vi "Add Data Type.vi"(7 "Control Info Cluster in":T1, 8 "error in (no error)":errorcluster, 10 "Data Type String":string, 11 "Control in":refnum<vi>) -> (0 "error out":errorcluster, 2 "TypeDef?":bool, 3 "Control out":refnum<vi>, 5 "Control Info Cluster out":T1)   [LabVIEW 2023, in "VIDoc Parsing.lvlib"]
doc: "Adds Data Type String to the Control Info Cluster, handing Typedefs specially."
uses:
  VIDoc Parsing.lvlib
  TypeDefs/Controls Info Cluster.ctl
  <vilib>/picture/picture.llb/imagedata.ctl
  <vilib>/Utility/miscctls.llb/LVKeyTypeDef.ctl
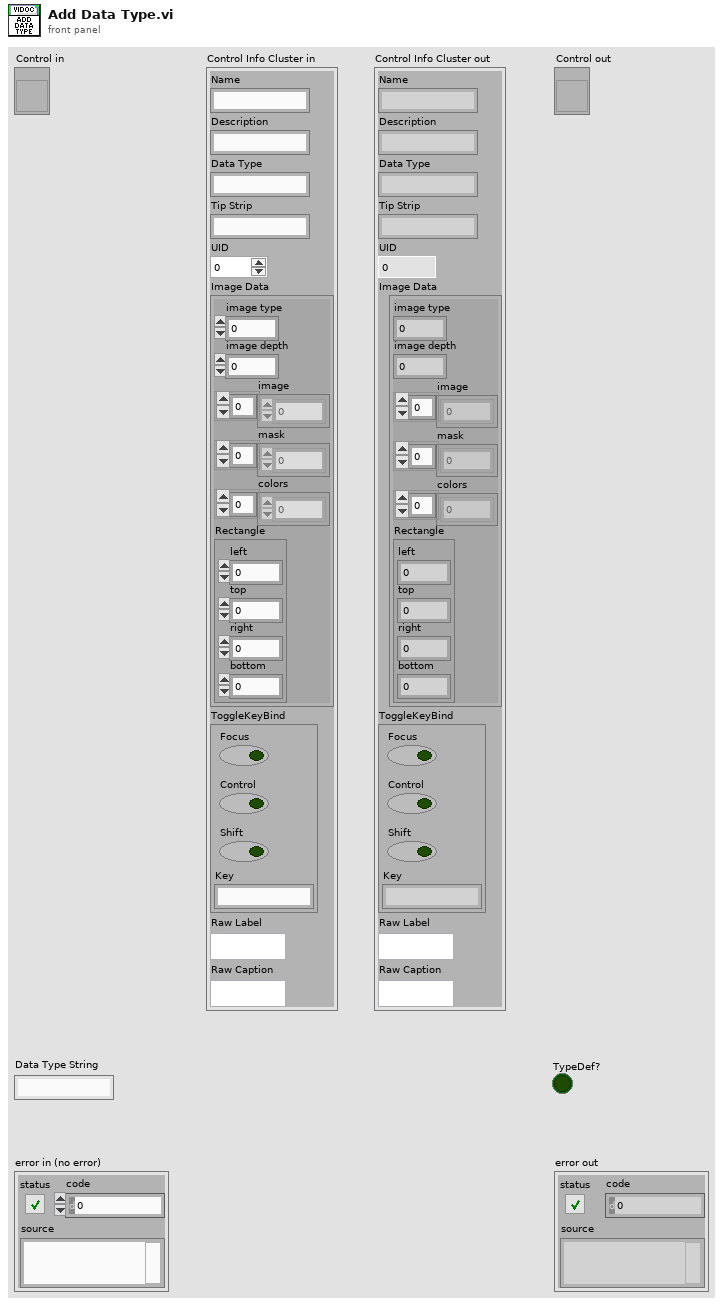
[diagram p1: front panel]
types:
  T1 = typedef "VIDoc Parsing.lvlib/Controls Info Cluster.ctl" = cluster{"Name":string, "Description":string, "Data Type":string, "Tip Strip":string, "UID":i32, "Image Data":T2, "ToggleKeyBind":T3, "Raw Label":string, "Raw Caption":string}
  T2 = typedef "imagedata.ctl" = cluster{"image type":i32, "image depth":i32, "image":u8[], "mask":u8[], "colors":u32[], "Rectangle":cluster{"left":i16, "top":i16, "right":i16, "bottom":i16}}
  T3 = typedef "LVKeyTypeDef.ctl" = cluster{"Focus":bool, "Control":bool, "Shift":bool, "Key":string}
  T4 = enum32{"not a typedef", "typedef", "strict typedef", "class private data"}
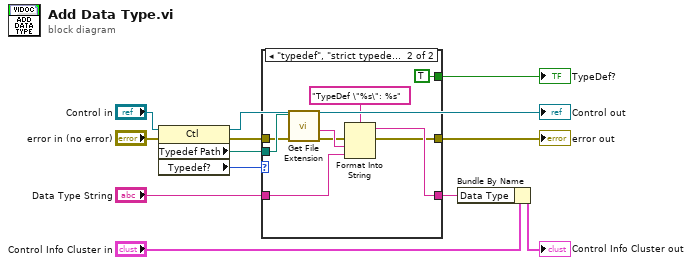
[diagram p0: block diagram]
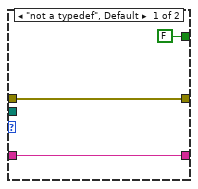
[diagram p2: hidden frame]
diagram:
  n1 = property class="Ctl"(reference="Control in", error in="error in (no error)") -> (reference out=→"Control out":refnum<vi>, error out=w6:errorcluster, "Typedef Path"=w8:path, "Typedef?"=w7:T4)
  n2 = case shown="\"typedef\", \"strict typedef\"" w7 {
    tunnel: w8 -> [_ w24]
    tunnel: "Data Type String" -> [w15 w23]
    tunnel: [w15 w22] -> w3
    tunnel: w6 -> [w14 w18]
    tunnel: [w14 w17] -> w2
    tunnel: [FALSE TRUE] -> w1
    frame "not a typedef", Default {
    }
    frame "typedef", "strict typedef" {
      n3 = call <vilib>:"Get File Extension.vi"("error in (no error)"=w18, "file"=w24) -> ("error out"=w19:errorcluster, "filename without extension"=w20:string)  [unwired: 5 in, 3 out]
      n4 = Format Into String(format string="TypeDef \"%s\": %s", error in=w19, w20, w23) -> (resulting string=w22:string, error out=w17:errorcluster)  [unwired: 1 in]
    }
  }
  "error out" <- w2
  "TypeDef?" <- w1
  n5 = Bundle By Name(cluster="Control Info Cluster in", "Data Type"=w3) -> (→"Control Info Cluster out":T1)
